vi "Build Prompt.vi"(8 "error in (no error)":errorcluster, 10 "Prompt text":string="What object do you see on the attached image.", 11 "path to JPEG file":path=path "C:/batt/IMG_3307.jpg") -> (0 "error out":errorcluster, 3 "Prompt":string)   [LabVIEW 2025, in "Battery Prompt.lvlib"]
doc: "Build a GPT prompt in a form required by the OpenAI API. Uses string replacement to join the JSONs as the items of the request array are not homogenious."
uses:
  Battery Prompt.lvlib
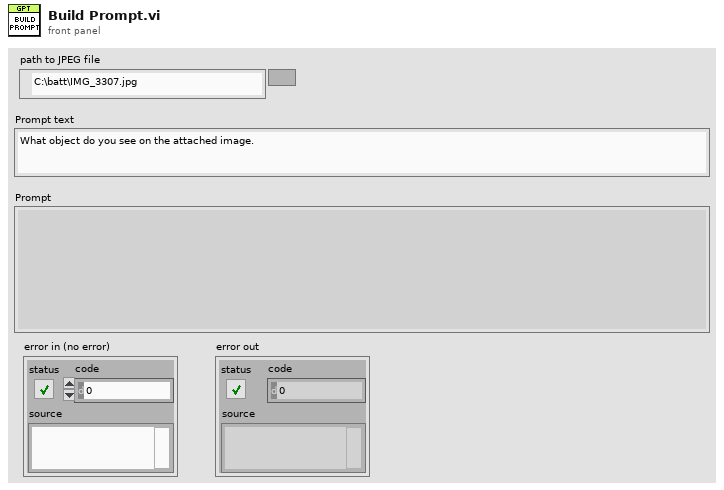
[diagram p1: front panel]
types:
  T1 = cluster{"type":string, "image_url":cluster{"url":string}}
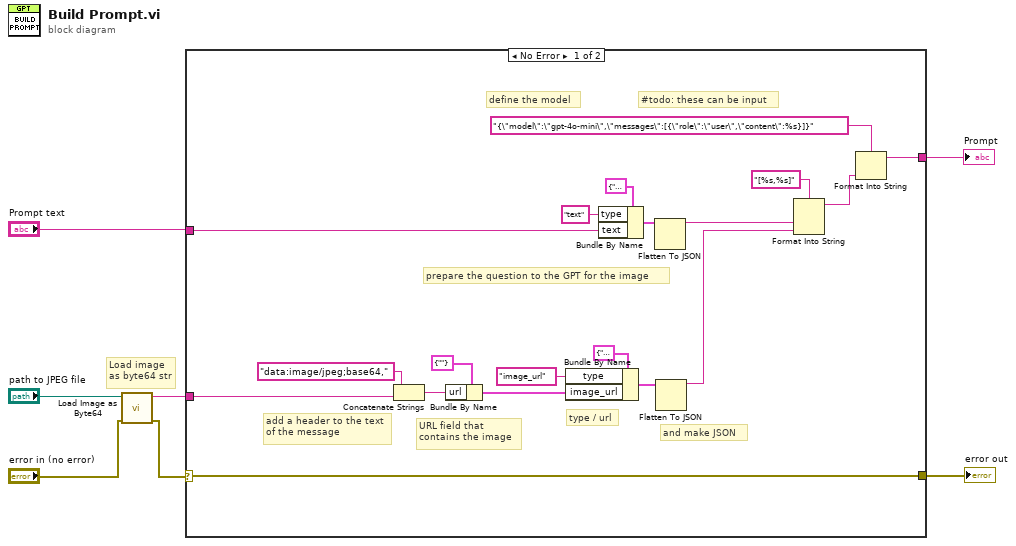
[diagram p0: block diagram]
diagram:
  # "Load image \nas byte64 str"
  n1 = call "Load Image as Byte64.vi"("error in (no error)"="error in (no error)", "path to JPEG file"="path to JPEG file") -> ("error out"=w2:errorcluster, "Image String"=w6:string)  [unwired: 8 in]
  n2 = case shown="No Error" w2 {
    selector: w2 -> [w9 w27]
    tunnel: [w11 _] -> w7
    tunnel: w6 -> [w10 _]
    tunnel: [w9 w27] -> w5
    tunnel: "Prompt text" -> [w8 _]
    frame No Error {
      # "#todo: these can be input"
      # "define the model"
      # "prepare the question to the GPT for the image"
      # "and make JSON"
      # "type / url"
      # "URL field that\ncontains the image"
      # "add a header to the text\nof the message"
      n3 = Concatenate Strings("data:image/jpeg;base64,", w10) -> (w23:string)
      n4 = Bundle By Name(cluster=cluster{"url":string} {"url"=""}, "url"=w23) -> (w22:cluster{"url":string})
      n5 = Bundle By Name(cluster=T1 {"type"="", "image_url"={"url"=""}}, "type"="image_url", "image_url"=w22) -> (w17:T1)
      n6 = Bundle By Name(cluster=cluster{"type":string, "text":string} {"type"="", "text"=""}, "type"="text", "text"=w8) -> (w18:cluster{"type":string, "text":string})
      n7 = Flatten To JSON(anything=w18) -> (JSON string=w14:string)  [unwired: 2 in, 1 out]
      n8 = Flatten To JSON(anything=w17) -> (JSON string=w13:string)  [unwired: 2 in, 1 out]
      n9 = Format Into String(format string="[%s,%s]", w14, w13) -> (resulting string=w12:string)  [unwired: 2 in, 1 out]
      n10 = Format Into String(format string="{\"model\":\"gpt-4o-mini\",\"messages\":[{\"role\":\"user\",\"content\":%s}]}", w12) -> (resulting string=w11:string)  [unwired: 2 in, 1 out]
    }
    frame Error {
    }
  }
  "Prompt" <- w7
  "error out" <- w5
